vi "Test Weighted Stimulus Synthesis.vi"() -> ()   [LabVIEW 2015]
uses:
  Type Defs/Cal Stimulus.ctl
  Type Defs/ACal-Multiband Parameters.ctl
  Utility VIs/Type Defs/Speaker ring.ctl
  Utility VIs/Math VIs/FFT x(t) to dB,Degrees (1D).vi
panel:
  out "XY Graph":T1(graph)
  out "Waveform Graph":dbl[](graph)
  in  "Speaker":T2
  in  "Weighted":T3={"Folder"=path "D:/Data/Chamber 1 Calibration", "Fmin"=4000.0, "Fmax"=45000.0, "Max range"=30.0, "WF"=0} {"WF" items=["Chirp", "Noise"]}
  in  "Cal Stimulus":T4={"Min Freq (Hz)"=4000.0, "Max Freq (Hz)"=45000.0, "Freq Step (Hz)"=50.0, "Waveform"=enum."Chirp", "Attenuation (dB)"=0.0, "Sample Rate (Hz)"=100000.0}
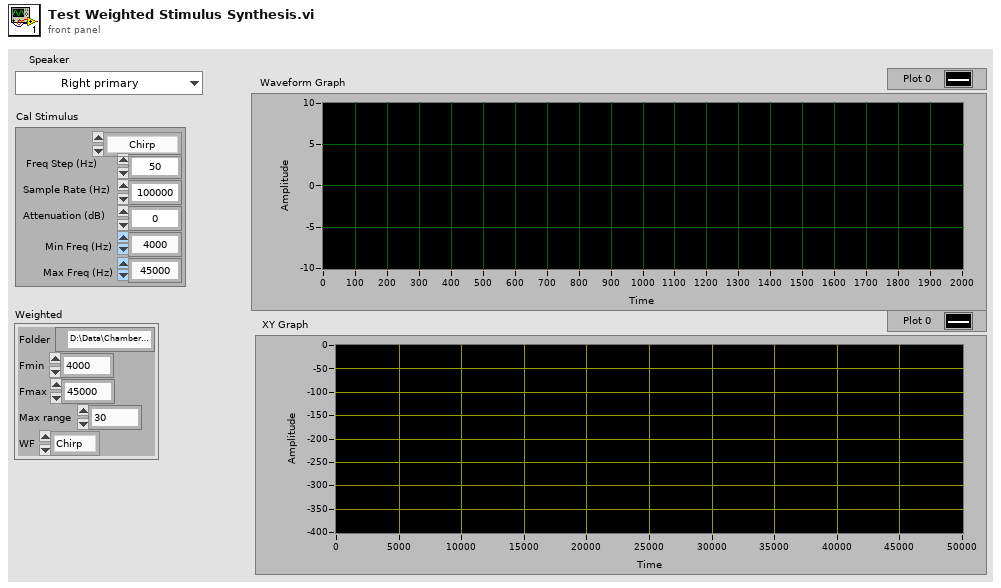
[diagram p1: front panel]
types:
  T1 = cluster{"Freq (Hz)":dbl[], "+Freq. Mag of FFT (dB rms)":dbl[]}
  T2 = typedef "Speaker ring.ctl" = enum16{"Right primary", "Right secondary", "Left primary", "Left secondary"}
  T3 = typedef "ACal-Multiband Parameters.ctl" = cluster{"Folder":path, "Fmin":dbl, "Fmax":dbl, "Max range":dbl, "WF":u16}
  T4 = typedef "Cal Stimulus.ctl" = cluster{"Min Freq (Hz)":dbl, "Max Freq (Hz)":dbl, "Freq Step (Hz)":dbl, "Waveform":enum16{"Chirp", "Weighted"}, "Attenuation (dB)":dbl, "Sample Rate (Hz)":dbl}
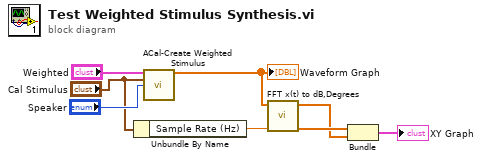
[diagram p0: block diagram]
diagram:
  n1 = Unbundle By Name("Cal Stimulus") -> ("Sample Rate (Hz)"=w1:dbl)
  n2 = call "ACal-Create Weighted Stimulus.vi"("Weighted"="Weighted", "Cal Stimulus"="Cal Stimulus", "Speaker"="Speaker") -> ("Stimulus"=w6:dbl[])  [unwired: 11 in, 1 out]
  "Waveform Graph" <- w6
  n3 = call-poly "FFT x(t) to dB,Degrees.vi"("Fs (Hz)"=w1, "X"=w6) -> ("Freq (Hz)"=w5:dbl[], "+Freq. Mag of FFT (dB rms)"=w4:dbl[])  [unwired: 7 in, 1 out]
  n4 = Bundle("Freq (Hz)"=w5, "+Freq. Mag of FFT (dB rms)"=w4) -> (→"XY Graph":T1)  [unwired: 1 in]
